vi "Gear_Placer_OperatorAssist.vi"(0 "Start?":bool, 1 "Reset?":bool, 2 "Ultrasonic":dbl=-1.5822026199325805, 3 "Rail_Finished?":bool=TRUE, 4 "Gate_Finished?":bool=TRUE, 5 "Gear_Pusher_Finished?":bool=TRUE, 6 "Gear_Orientation_Offset_In":dbl=1.0, 7 "Place_Gear?":bool, 8 "RailTargetClamp":dbl=6.5, 9 "Gear_Orientation_Bb_True?":bool, 10 "GearMiddleOffset":dbl) -> (11 "Returning":bool=TRUE, 12 "Gear_Orientation_Offset_Out":dbl, 13 "Place_Complete?":bool=TRUE, 14 "Rail_Track?":bool, 15 "Rail_Target_Position":dbl=30.0, 16 "Gate_Pos":T1, 17 "Gear_Pusher_Extend?":bool, 18 "Gear_Chute_Extend?":bool, 19 "State":T2)   [LabVIEW 2016]
uses:
  TypeDefs/GearPlaceState_Type.ctl
  TypeDefs/GatePos_Type.ctl
  ArgosLib/Signal Processing/TypeDefs/EdgeDetector_Type.ctl
  Global_Var-RefNum/Global_Var_Other.vi
  Global_Var-RefNum/Global_Var_Drive.vi
  ArgosLib/ArgosLib.lvlib
panel:
  out "s? t:f":dbl
  in  "P":dbl=0.2 format="%#_13g"
  in  "middle":dbl=15.0 format="%#_13g"
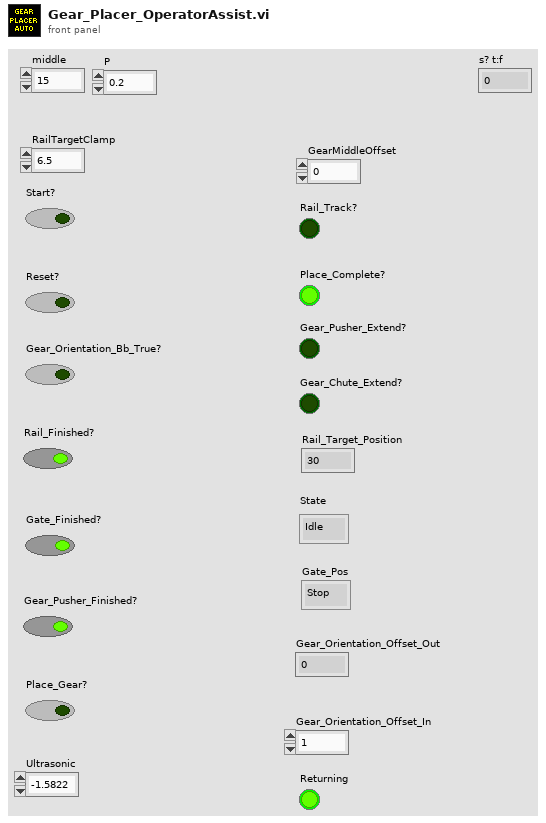
[diagram p1: front panel]
types:
  T1 = typedef "GatePos_Type.ctl" = enum16{"Stop", "Catch", "Clamp", "Open"}
  T2 = typedef "GearPlaceState_Type.ctl" = enum16{"Idle", "Wait for Peg", "Allign To Lift", "Arm Gear", "Place Gear", "Return to Ready", "Disarm Gear"}
  T3 = typedef "EdgeDetector_Type.ctl" = enum16{"RisingEdge", "FallingEdge", "Both"}
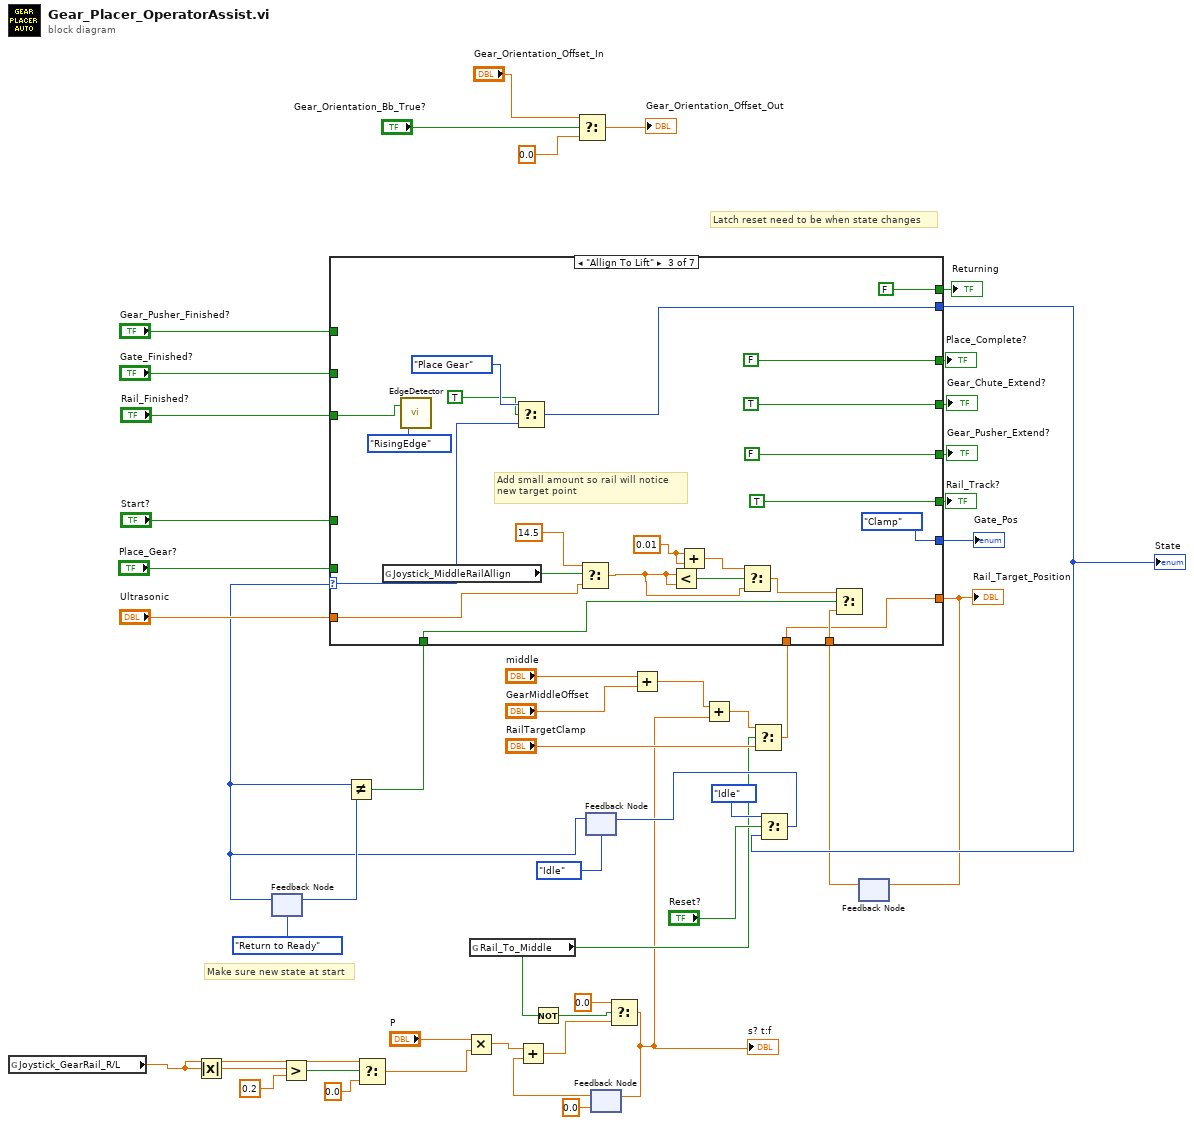
[diagram p0: block diagram]
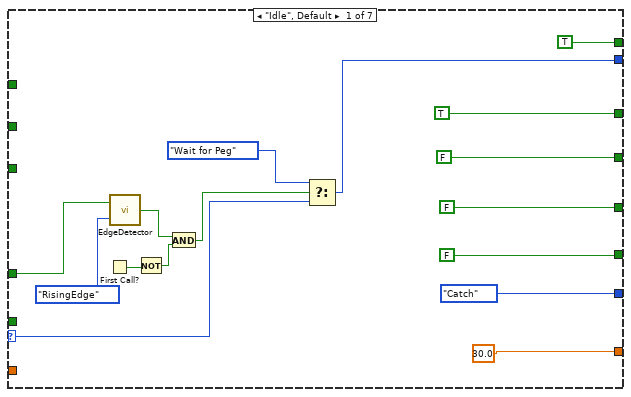
[diagram p2: hidden frame]
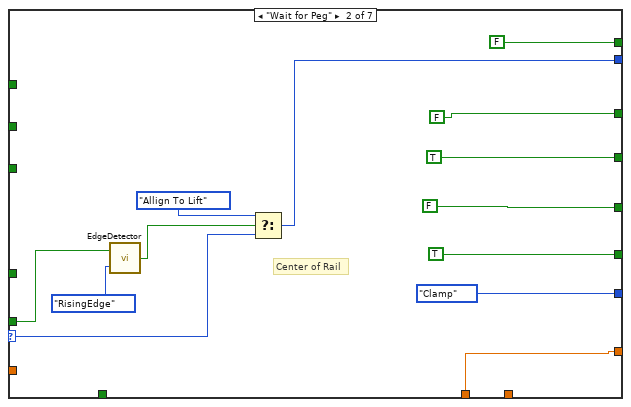
[diagram p3: hidden frame]
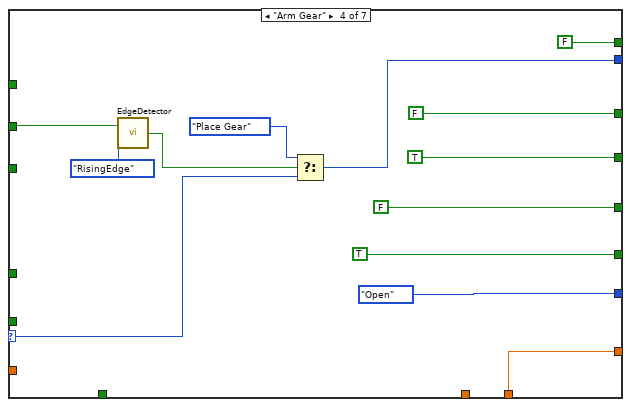
[diagram p4: hidden frame]
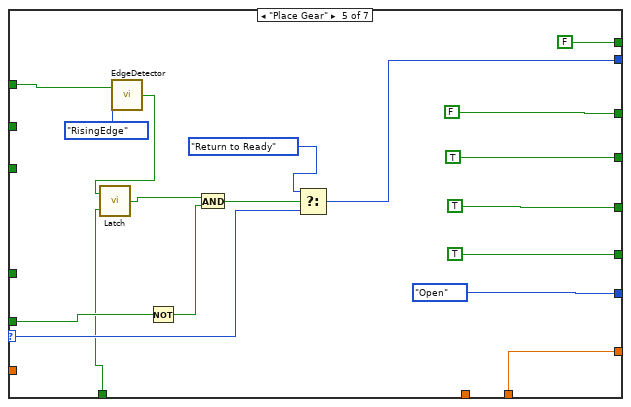
[diagram p5: hidden frame]
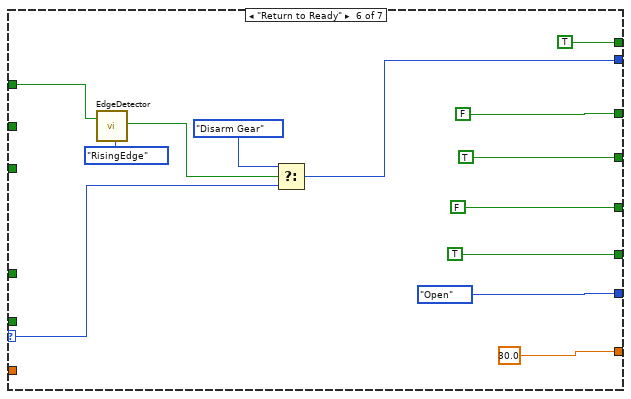
[diagram p6: hidden frame]
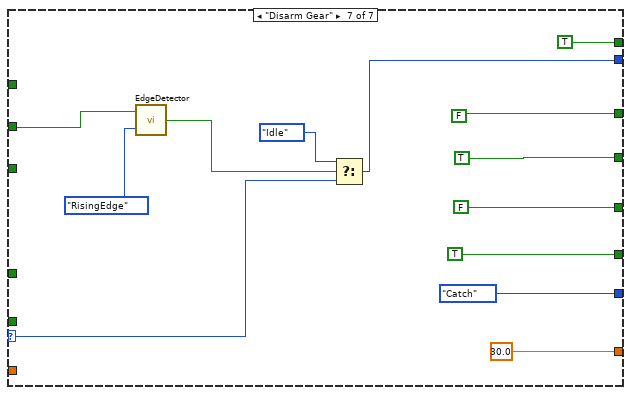
[diagram p7: hidden frame]
diagram:
  # "Make sure new state at start"
  # "Latch reset need to be when state changes"
  n1 = global read "Global_Var_Drive.vi" "Joystick_GearRail_R/L"() -> (w4:dbl)
  n2 = Absolute Value(x=w4) -> (abs(x)=w11:dbl)
  n3 = feedback #1(GearPlaceState_Type."Return to Ready") -> (w31:T2)
  n4 = Greater?(x=w11, y=0.2) -> (0:w9:bool)
  n5 = Select(t=w4, s=w9, f=0.0) -> (s? t:f=w3:dbl)
  n6 = Multiply(x="P", y=w3) -> (x*y=w15:dbl)
  n7 = global read "Global_Var_Other.vi" "Rail_To_Middle"() -> (w12:bool)
  n8 = Not(x=w12) -> (.not. x?=w13:bool)
  n9 = Select(t="Gear_Orientation_Offset_In", s="Gear_Orientation_Bb_True?", f=0.0) -> (s? t:f=→"Gear_Orientation_Offset_Out":dbl)
  n10 = feedback #2(GearPlaceState_Type."Idle") -> (w24:T2)
  n11 = feedback-in #1(w24) -> ()
  n12 = Not Equal?(x=w24, y=w31) -> (x != y?=w38:bool)
  n13 = feedback #3(0.0) -> (w18:dbl)
  n14 = Add(x=w15, y=w18) -> (x+y=w19:dbl)
  n15 = Select(t=0.0, s=w13, f=w19) -> (s? t:f=w5:dbl)
  "s? t:f" <- w5
  n16 = feedback-in #3(w5) -> ()
  n17 = Add(x="middle", y="GearMiddleOffset") -> (x+y=w2:dbl)
  n18 = Add(x=w2, y=w5) -> (x+y=w6:dbl)
  n19 = Select(t=w6, s=w12, f="RailTargetClamp") -> (s? t:f=w21:dbl)
  n20 = feedback #4() -> (w32:dbl)  [unwired: 1 in]
  n21 = case shown="\"Allign To Lift\"" w24 {
    selector: w24 -> [w61 w74 w92 w110 w127 w141 w154]
    tunnel: [w64 w76 w91 w112 w129 w143 w156] -> w40
    tunnel: "Rail_Finished?" -> [_ _ w98 _ _ _ _]
    tunnel: "Gate_Finished?" -> [_ _ _ w108 _ _ w153]
    tunnel: "Start?" -> [w56 _ _ _ _ _ _]
    tunnel: "Gear_Pusher_Finished?" -> [_ _ _ _ w122 w139 _]
    tunnel: [FALSE TRUE TRUE TRUE TRUE TRUE TRUE] -> w41
    tunnel: "Place_Gear?" -> [_ w70 _ _ w125 _ _]
    tunnel: w38 -> [_ _ w90 _ w120 _ _]
    tunnel: [GatePos_Type."Catch" ("Gate_Pos") GatePos_Type."Clamp" ("Gate_Pos") GatePos_Type."Clamp" ("Gate_Pos") GatePos_Type."Open" ("Gate_Pos") GatePos_Type."Open" ("Gate_Pos") GatePos_Type."Open" ("Gate_Pos") GatePos_Type."Catch" ("Gate_Pos")] -> w37
    tunnel: [FALSE FALSE FALSE FALSE TRUE FALSE FALSE] -> w36
    tunnel: [FALSE TRUE TRUE TRUE TRUE TRUE TRUE] -> w35
    tunnel: "Ultrasonic" -> [_ _ w87 _ _ _ _]
    tunnel: [30.0 w65 w81 w103 w116 30.0 30.0] -> w33
    tunnel: w32 -> [_ _ w93 w103 w116 _ _]
    tunnel: [TRUE FALSE FALSE FALSE FALSE FALSE FALSE] -> w30
    tunnel: [TRUE FALSE FALSE FALSE FALSE TRUE TRUE] -> w22
    tunnel: w21 -> [_ w65 w81 _ _ _ _]
    frame "Idle", Default {
      n22 = First Call?() -> (First Call?: T/F=w52:bool)
      n23 = call "EdgeDetector.vi"("DetectorType"=EdgeDetector_Type."RisingEdge", "Input"=w56) -> ("Edge"=w53:bool)
      n24 = Not(x=w52) -> (.not. x?=w54:bool)
      n25 = And(x=w53, y=w54) -> (x .and. y?=w51:bool)
      n26 = Select(t=GearPlaceState_Type."Wait for Peg", s=w51, f=w61) -> (s? t:f=w64:T2)
    }
    frame "Wait for Peg" {
      # "Center of Rail"
      n27 = call "EdgeDetector.vi"("DetectorType"=EdgeDetector_Type."RisingEdge", "Input"=w70) -> ("Edge"=w68:bool)
      n28 = Select(t=GearPlaceState_Type."Allign To Lift", s=w68, f=w74) -> (s? t:f=w76:T2)
    }
    frame "Allign To Lift" {
      w79 = 0.01 ("x")
      # "Add small amount so rail will notice\nnew target point"
      n29 = global read "Global_Var_Drive.vi" "Joystick_MiddleRailAllign"() -> (w86:bool)
      n30 = call "EdgeDetector.vi"("DetectorType"=EdgeDetector_Type."RisingEdge", "Input"=w98) -> ()  [unwired: 1 out]
      n31 = Select(t=GearPlaceState_Type."Place Gear", s=TRUE, f=w92) -> (s? t:f=w91:T2)
      n32 = Select(t=14.5, s=w86, f=w87) -> (s? t:f=w80:dbl)
      n33 = Less?(x=w80, y=w80) -> (x < y?=w84:bool)
      n34 = Add(x=w79, y=w79) -> (x+y=w82:dbl)
      n35 = Select(t=w82, s=w84, f=w80) -> (s? t:f=w83:dbl)
      n36 = Select(t=w83, s=w90, f=w93) -> ()  [unwired: 1 out]
    }
    frame "Arm Gear" {
      n37 = call "EdgeDetector.vi"("DetectorType"=EdgeDetector_Type."RisingEdge", "Input"=w108) -> ("Edge"=w109:bool)
      n38 = Select(t=GearPlaceState_Type."Place Gear", s=w109, f=w110) -> (s? t:f=w112:T2)
    }
    frame "Place Gear" {
      n39 = call "EdgeDetector.vi"("DetectorType"=EdgeDetector_Type."RisingEdge", "Input"=w122) -> ("Edge"=w121:bool)
      n40 = call "Latch.vi"("Reset"=w120, "Input"=w121) -> ("LatchOut"=w123:bool)
      n41 = Not(x=w125) -> (.not. x?=w126:bool)
      n42 = And(x=w123, y=w126) -> (x .and. y?=w131:bool)
      n43 = Select(t=GearPlaceState_Type."Return to Ready", s=w131, f=w127) -> (s? t:f=w129:T2)
    }
    frame "Return to Ready" {
      n44 = call "EdgeDetector.vi"("DetectorType"=EdgeDetector_Type."RisingEdge", "Input"=w139) -> ("Edge"=w140:bool)
      n45 = Select(t=GearPlaceState_Type."Disarm Gear", s=w140, f=w141) -> (s? t:f=w143:T2)
    }
    frame "Disarm Gear" {
      n46 = call "EdgeDetector.vi"("DetectorType"=EdgeDetector_Type."RisingEdge", "Input"=w153) -> ("Edge"=w148:bool)
      n47 = Select(t=GearPlaceState_Type."Idle", s=w148, f=w154) -> (s? t:f=w156:T2)
    }
  }
  "Rail_Track?" <- w41
  "State" <- w40
  "Gate_Pos" <- w37
  "Gear_Pusher_Extend?" <- w36
  "Gear_Chute_Extend?" <- w35
  "Rail_Target_Position" <- w33
  "Place_Complete?" <- w30
  "Returning" <- w22
  n48 = Select(t=GearPlaceState_Type."Idle", s="Reset?", f=w40) -> (s? t:f=w23:T2)
  n49 = feedback-in #2(w23) -> ()
  n50 = feedback-in #4(w33) -> ()
